vi "EditMeasurement.vi"(7 "reference measure":sgl, 8 "error in (no error)":errorcluster, 9 "instrument measure":sgl, 10 "measurement-id":u16, 11 "ByteGSAPIBase in":refnum<class "ByteGSAPIBase.lvclass">) -> (0 "error out":errorcluster, 2 "measurement data":T1, 3 "ByteGSAPIBase out":refnum<class "ByteGSAPIBase.lvclass">)   [LabVIEW 2019, in "ByteGSWebAPI.lvlib" / "ByteGSAPIBase.lvclass"]
doc: "Edit a measurement based on the measurement-id"
uses:
  ByteGSAPIBase.lvclass
  MeasurementResData.ctl
  <vilib>/Bytelabs/ByteREST/ByteRESTClass/ByteRESTBase/HTTP/Status_Code.ctl
  TypeDef/EditMeasurementReqData.ctl
  ByteGSAPIBase.lvclass/ByteGSAPIBase.ctl
  <vilib>/Bytelabs/ByteREST/ByteRESTClass/ByteRESTBase/RESTBase.lvclass
  <vilib>/numeric/Random Number (Range) U64.vi
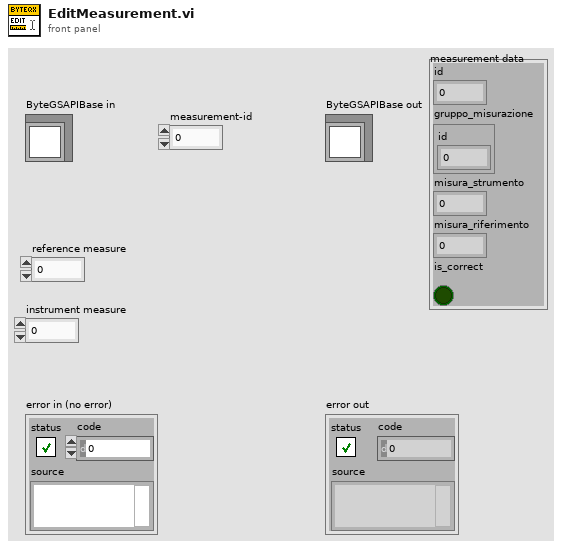
[diagram p1: front panel]
types:
  T1 = typedef "ByteGSWebAPI.lvlib/ByteGSAPIBase.lvclass/MeasurementResData.ctl" = cluster{"id":i32, "gruppo_misurazione":cluster{"id":i32}, "misura_strumento":dbl, "misura_riferimento":dbl, "is_correct":bool}
  T2 = typedef "ByteGSWebAPI.lvlib/ByteGSAPIBase.lvclass/EditMeasurementReqData.ctl" = cluster{"Id_Group":i32, "misura_strumento":sgl, "misura_riferimento":sgl}
  T3 = typedef "ByteREST.lvlib/RESTBase.lvclass/Status_Code.ctl" = u16
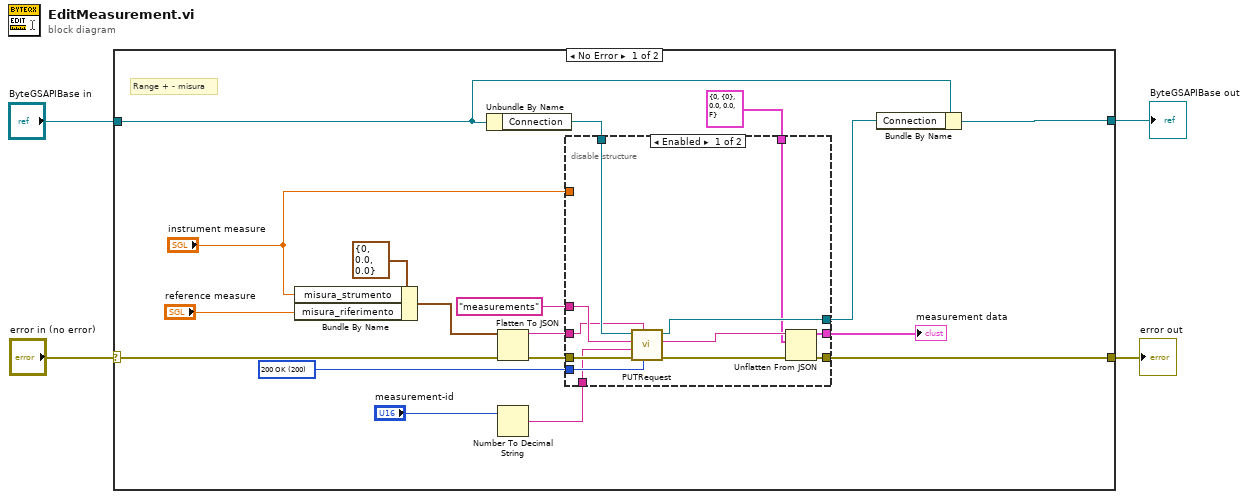
[diagram p0: block diagram]
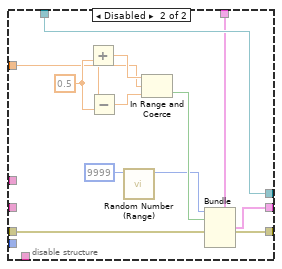
[diagram p2: hidden frame]
diagram:
  n1 = case shown="No Error" "error in (no error)" {
    selector: "error in (no error)" -> [w15 w48]
    tunnel: [w10 w48] -> w3
    tunnel: [w20 w47] -> w1
    tunnel: "ByteGSAPIBase in" -> [w22 w47]
    frame No Error {
      w17 = T3 200 items=["200 OK"=200, "201 Created"=201, "400 Bad Request"=400, "401 Unauthorized"=401, "403 Forbidden"=403, "404 Not Found"=404, "405 Method Not Allowed"=405, "406 Not Acceptable"=406, "500 Internal Server Error"=500] ("expected response")
      # "Range + - misura"
      n2 = Bundle By Name(cluster=T2 {"Id_Group"=0, "misura_strumento"=0.0, "misura_riferimento"=0.0} ("Valori"), "misura_strumento"="instrument measure", "misura_riferimento"="reference measure") -> (w13:T2)
      n3 = Unbundle By Name(w22) -> ("Connection"=w21:refnum<class "RESTBase.lvclass">)
      n4 = Flatten To JSON(anything=w13, error in (no error)=w15) -> (JSON string=w12:string, 11:w14:errorcluster)  [unwired: 1 in]
      n5 = Number To Decimal String(number="measurement-id") -> (decimal integer string=w7:string)  [unwired: 1 in]
      n6 = disable-structure shown="Enabled" {
        disable-tunnel: w21 -> [w34 w39]
        disable-tunnel: [w33 w39] -> w19
        disable-tunnel: "measurements" ("Request") -> [w32 _]
        disable-tunnel: w17 -> [w31 _]
        disable-tunnel: w14 -> [w30 w35]
        disable-tunnel: w12 -> [w29 _]
        disable-tunnel: T1 {"id"=0, "gruppo_misurazione"={"id"=0}, "misura_strumento"=0.0, "misura_riferimento"=0.0, "is_correct"=FALSE} -> [w26 w37]
        disable-tunnel: [w25 w41] -> w6
        disable-tunnel: [w24 w35] -> w10
        disable-tunnel: "instrument measure" -> [_ w43]
        disable-tunnel: w7 -> [w23 _]
        frame Enabled {
          n7 = call-dynamic "PUTRequest.vi"("expected response"=w31, "Body in"=w29, "error in (no error)"=w30, "Parameter"=w23, "Request"=w32, "ByteRESTBase in"=w34) -> ("error out"=w27:errorcluster, "Body"=w28:string, "ByteRESTBase out"=w33:refnum<class "RESTBase.lvclass">)  [unwired: 2 in, 1 out]
          n8 = Unflatten From JSON(JSON string=w28, type and defaults=w26, error in (no error)=w27) -> (value=w25:T1, error out=w24:errorcluster)  [unwired: 4 in]
        }
        frame Disabled {
          w44 = 0.5
          n9 = Subtract(y=w44) -> (x=w42:dbl, x-y=w46:dbl)
          n10 = Add(x=w42, y=w44) -> (x+y=w45:dbl)
          n11 = call-poly <vilib>:"Random Number (Range).vi"("upper bound (100)"=u64 9999) -> ("number"=w36:u64)  [unwired: 10 in]
          n12 = In Range and Coerce(upper limit=w45, x=w43, lower limit=w46) -> (In Range?=w40:bool)  [unwired: 1 out]
          n13 = Bundle(cluster=w37, "id"=w36, "gruppo_misurazione"=w40) -> (w41:T1)  [unwired: 3 in]
        }
      }
      "measurement data" <- w6
      n14 = Bundle By Name(cluster=w22, "Connection"=w19) -> (w20:refnum<class "ByteGSAPIBase.lvclass">)
    }
    frame Error {
    }
  }
  "error out" <- w3
  "ByteGSAPIBase out" <- w1
